vi "4155C 1D-2D array.vi"(4 "Number of VAR1 steps":i32, 5 "1D array in":dbl[](array[numeric]) format="%.2f") -> (1 "2D array out":dbl[][](array[numeric]) format="%.2f")   [LabVIEW 2016]
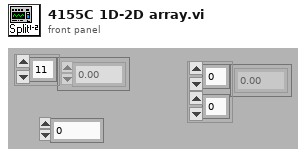
[diagram p1: front panel]
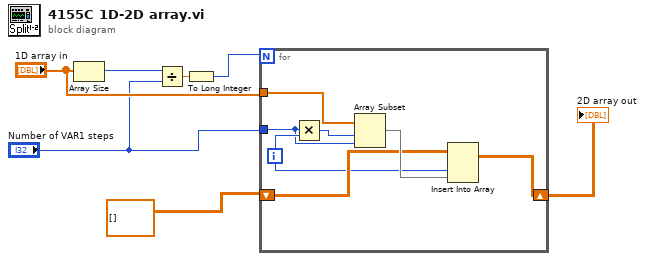
[diagram p0: block diagram]
diagram:
  n1 = Array Size(array="1D array in") -> (size(s)=w4:i32)
  n2 = Divide(x=w4, y="Number of VAR1 steps") -> (x/y=w7:dbl)
  n3 = To Long Integer(number=w7) -> (32bit integer=w2:i32)
  n4 = for {
    N: w2 -> [_]
    tunnel: "Number of VAR1 steps" -> [w8]
    tunnel: "1D array in" -> [w13]
    shift-right: [w9] -> w5
    shift-left: dbl[][] [] ("Array Constant") -> [w11]
    i -> [w10]
    n5 = Multiply(x=w8, y=w10) -> (x*y=w14:i32)
    n6 = Array Subset(array=w13, index=w14, length=w8) -> (w12:dbl[])
    n7 = Insert Into Array(array=w11, index (col)=w10, new element=w12) -> (w9:dbl[][])  [unwired: 1 in]
  }
  "2D array out" <- w5
